vi "Parse_Limit_File.vi"(8 "error in":errorcluster, 11 "file path (dialog if empty)":path) -> (0 "error out":errorcluster, 1 "IncorrectString":string, 2 "AllThresholds":T1={"TC0"={"Enable"=FALSE, "LoErr"=0.0, "LoWarn"=0.0, "HiWarn"=0.0, "HiErr"=0.0, "RX?"=TRUE}, "TC1"={"Enable"=FALSE, "LoErr"=0.0, "LoWarn"=0.0, "HiWarn"=0.0, "HiErr"=0.0, "RX?"=TRUE}, "TC2"={"Enable"=FALSE, "LoErr"=0.0, "LoWarn"=0.0, "HiWarn"=0.0, "HiErr"=0.0, "RX?"=TRUE}, "TC3"={"Enable"=FALSE, "LoErr"=0.0, "LoWarn"=0.0, "HiWarn"=0.0, "HiErr"=0.0, "RX?"=TRUE}, "TC4"={"Enable"=FALSE, "LoErr"=0.0, "LoWarn"=0.0, "HiWarn"=0.0, "HiErr"=0.0, "RX?"=TRUE}, "TC5"={"Enable"=FALSE, "LoErr"=0.0, "LoWarn"=0.0, "HiWarn"=0.0, "HiErr"=0.0, "RX?"=TRUE}, "TC6"={"Enable"=FALSE, "LoErr"=0.0, "LoWarn"=0.0, "HiWarn"=0.0, "HiErr"=0.0, "RX?"=TRUE}, "TC7"={"Enable"=FALSE, "LoErr"=0.0, "LoWarn"=0.0, "HiWarn"=0.0, "HiErr"=0.0, "RX?"=TRUE}, "TC8"={"Enable"=FALSE, "LoErr"=0.0, "LoWarn"=0.0, "HiWarn"=0.0, "HiErr"=0.0, "RX?"=TRUE}, "TC9"={"Enable"=FALSE, "LoErr"=0.0, "LoWarn"=0.0, "HiWarn"=0.0, "HiErr"=0.0, "RX?"=TRUE}, "TC10"={"Enable"=FALSE, "LoErr"=0.0, "LoWarn"=0.0, "HiWarn"=0.0, "HiErr"=0.0, "RX?"=TRUE}, "TC11"={"Enable"=FALSE, "LoErr"=0.0, "LoWarn"=0.0, "HiWarn"=0.0, "HiErr"=0.0, "RX?"=TRUE}, "TC12"={"Enable"=FALSE, "LoErr"=0.0, "LoWarn"=0.0, "HiWarn"=0.0, "HiErr"=0.0, "RX?"=TRUE}, "TC13"={"Enable"=FALSE, "LoErr"=0.0, "LoWarn"=0.0, "HiWarn"=0.0, "HiErr"=0.0, "RX?"=TRUE}, "TC14"={"Enable"=FALSE, "LoErr"=0.0, "LoWarn"=0.0, "HiWarn"=0.0, "HiErr"=0.0, "RX?"=TRUE}, "TC15"={"Enable"=FALSE, "LoErr"=0.0, "LoWarn"=0.0, "HiWarn"=0.0, "HiErr"=0.0, "RX?"=TRUE}, "TC16"={"Enable"=FALSE, "LoErr"=0.0, "LoWarn"=0.0, "HiWarn"=0.0, "HiErr"=0.0, "RX?"=TRUE}, "TC17"={"Enable"=FALSE, "LoErr"=0.0, "LoWarn"=0.0, "HiWarn"=0.0, "HiErr"=0.0, "RX?"=TRUE}, "TC18"={"Enable"=FALSE, "LoErr"=0.0, "LoWarn"=0.0, "HiWarn"=0.0, "HiErr"=0.0, "RX?"=TRUE}, "TC19"={"Enable"=FALSE, "LoErr"=0.0, "LoWarn"=0.0, "HiWarn"=0.0, "HiErr"=0.0, "RX?"=TRUE}, "TC20"={"Enable"=FALSE, "LoErr"=0.0, "LoWarn"=0.0, "HiWarn"=0.0, "HiErr"=0.0, "RX?"=TRUE}, "AI0"={"Enable"=FALSE, "LoErr"=0.0, "LoWarn"=0.0, "HiWarn"=0.0, "HiErr"=0.0, "RX?"=TRUE}, "AI1"={"Enable"=FALSE, "LoErr"=0.0, "LoWarn"=0.0, "HiWarn"=0.0, "HiErr"=0.0, "RX?"=TRUE}, "AI2"={"Enable"=FALSE, "LoErr"=0.0, "LoWarn"=0.0, "HiWarn"=0.0, "HiErr"=0.0, "RX?"=TRUE}, "AI3"={"Enable"=FALSE, "LoErr"=0.0, "LoWarn"=0.0, "HiWarn"=0.0, "HiErr"=0.0, "RX?"=TRUE}, "AI4"={"Enable"=FALSE, "LoErr"=0.0, "LoWarn"=0.0, "HiWarn"=0.0, "HiErr"=0.0, "RX?"=TRUE}, "AI5"={"Enable"=FALSE, "LoErr"=0.0, "LoWarn"=0.0, "HiWarn"=0.0, "HiErr"=0.0, "RX?"=TRUE}, "AI6"={"Enable"=FALSE, "LoErr"=0.0, "LoWarn"=0.0, "HiWarn"=0.0, "HiErr"=0.0, "RX?"=TRUE}, "AI7"={"Enable"=FALSE, "LoErr"=0.0, "LoWarn"=0.0, "HiWarn"=0.0, "HiErr"=0.0, "RX?"=TRUE}, "AI16"={"Enable"=FALSE, "LoErr"=0.0, "LoWarn"=0.0, "HiWarn"=0.0, "HiErr"=0.0, "RX?"=TRUE}, "AI17"={"Enable"=FALSE, "LoErr"=0.0, "LoWarn"=0.0, "HiWarn"=0.0, "HiErr"=0.0, "RX?"=TRUE}, "AI18"={"Enable"=FALSE, "LoErr"=0.0, "LoWarn"=0.0, "HiWarn"=0.0, "HiErr"=0.0, "RX?"=TRUE}, "AI19"={"Enable"=FALSE, "LoErr"=0.0, "LoWarn"=0.0, "HiWarn"=0.0, "HiErr"=0.0, "RX?"=TRUE}, "AI20"={"Enable"=FALSE, "LoErr"=0.0, "LoWarn"=0.0, "HiWarn"=0.0, "HiErr"=0.0, "RX?"=TRUE}, "AI21"={"Enable"=FALSE, "LoErr"=0.0, "LoWarn"=0.0, "HiWarn"=0.0, "HiErr"=0.0, "RX?"=TRUE}, "AI22"={"Enable"=FALSE, "LoErr"=0.0, "LoWarn"=0.0, "HiWarn"=0.0, "HiErr"=0.0, "RX?"=TRUE}, "AI23"={"Enable"=FALSE, "LoErr"=0.0, "LoWarn"=0.0, "HiWarn"=0.0, "HiErr"=0.0, "RX?"=TRUE}})   [LabVIEW 2018]
uses:
  Controls/Clusts/AllThresholds.ctl
  Controls/Clusts/ThresholdAlarmLimits.ctl
  <vilib>/Utility/file.llb/Read Delimited Spreadsheet (string).vi
  <vilib>/Utility/file.llb/Read Delimited Spreadsheet (DBL).vi
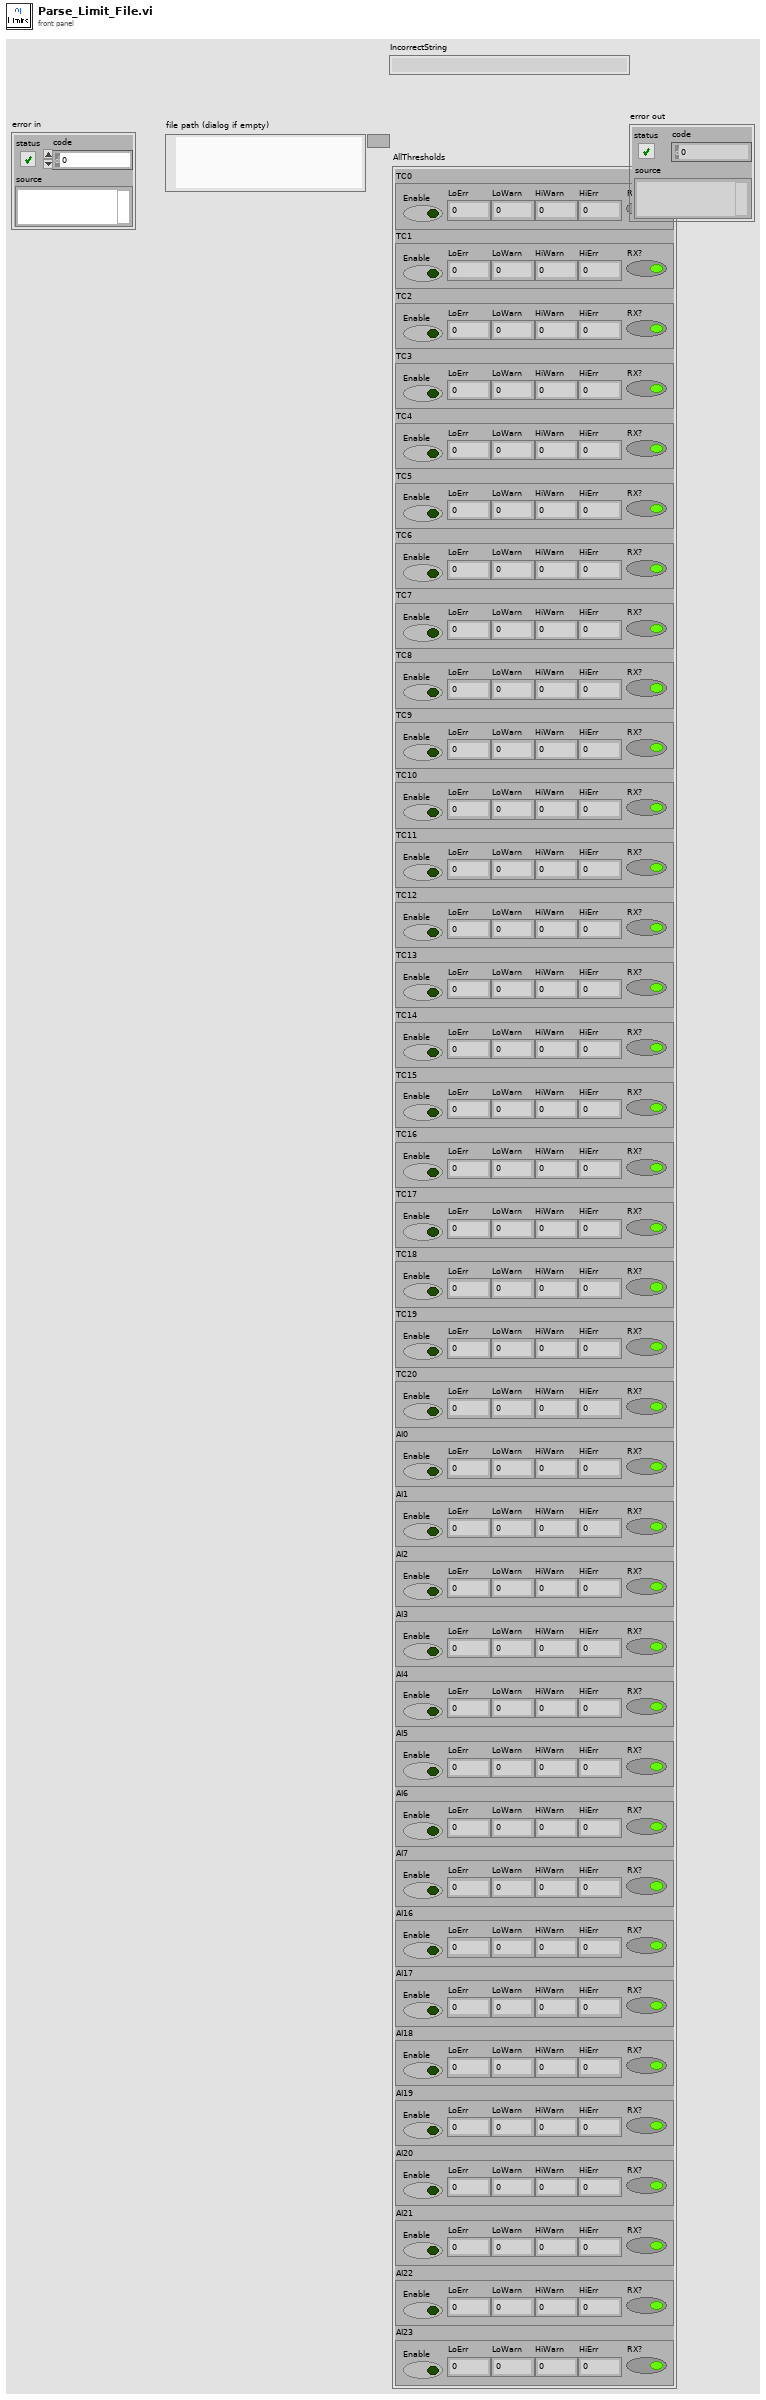
[diagram p1: front panel]
types:
  T1 = typedef "AllThresholds.ctl" = cluster{"TC0":T2, "TC1":T2, "TC2":T2, "TC3":T2, "TC4":T2, "TC5":T2, "TC6":T2, "TC7":T2, "TC8":T2, "TC9":T2, "TC10":T2, "TC11":T2, "TC12":T2, "TC13":T2, "TC14":T2, "TC15":T2, "TC16":T2, "TC17":T2, "TC18":T2, "TC19":T2, "TC20":T2, "AI0":T2, "AI1":T2, "AI2":T2, "AI3":T2, "AI4":T2, "AI5":T2, "AI6":T2, "AI7":T2, "AI16":T2, "AI17":T2, "AI18":T2, "AI19":T2, "AI20":T2, "AI21":T2, "AI22":T2, "AI23":T2}
  T2 = typedef "ThresholdAlarmLimits.ctl" = cluster{"Enable":bool, "LoErr":dbl, "LoWarn":dbl, "HiWarn":dbl, "HiErr":dbl, "RX?":bool}
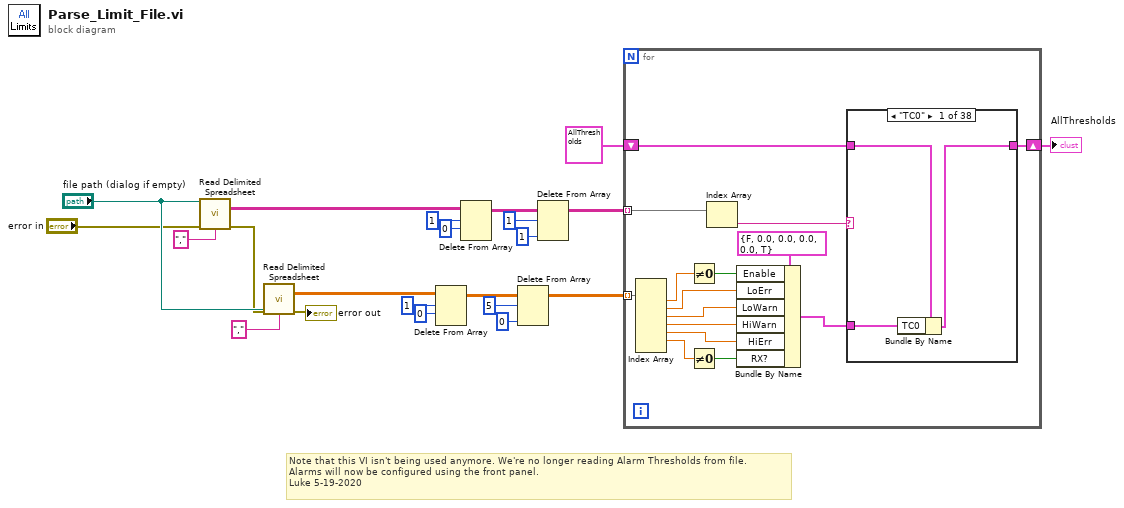
[diagram p0: block diagram]
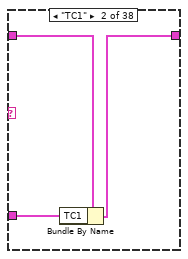
[diagram p2: hidden frame]
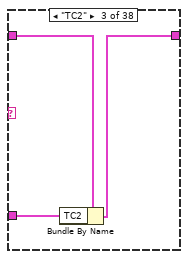
[diagram p3: hidden frame]
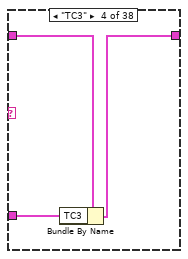
[diagram p4: hidden frame]
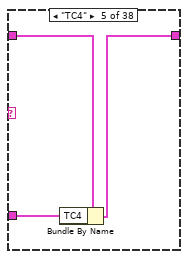
[diagram p5: hidden frame]
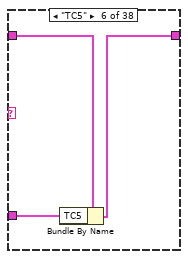
[diagram p6: hidden frame]
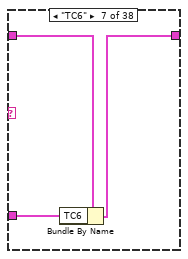
[diagram p7: hidden frame]
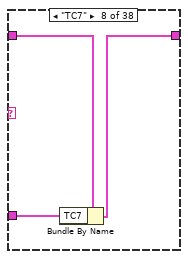
[diagram p8: hidden frame]
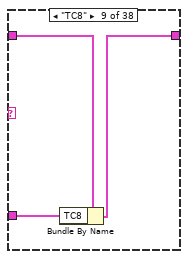
[diagram p9: hidden frame]
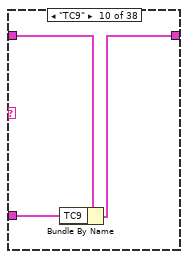
[diagram p10: hidden frame]
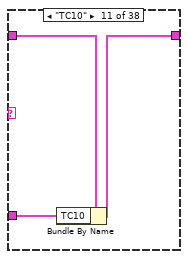
[diagram p11: hidden frame]
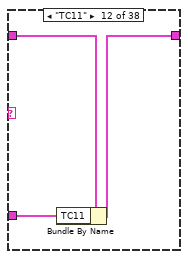
[diagram p12: hidden frame]
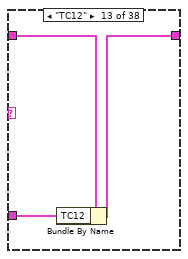
[diagram p13: hidden frame]
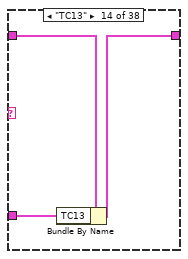
[diagram p14: hidden frame]
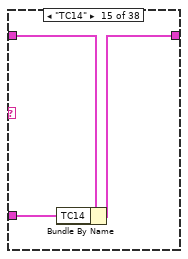
[diagram p15: hidden frame]
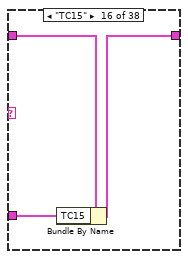
[diagram p16: hidden frame]
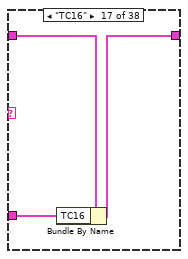
[diagram p17: hidden frame]
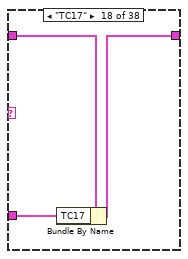
[diagram p18: hidden frame]
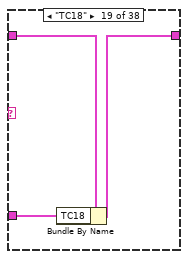
[diagram p19: hidden frame]
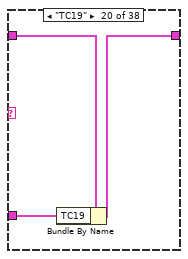
[diagram p20: hidden frame]
diagram:
  # "Note that this VI isn't being used anymore. We're no longer reading Alarm Thresholds from file.\nAlarms will now be configured using the front panel.\nLuke 5-19-2020"
  n1 = call-poly <vilib>:"Read Delimited Spreadsheet.vi"("file path (dialog if empty)"="file path (dialog if empty)", "error in (no error)"="error in", "delimiter (\\t)"="," ("delimiter (\\t)")) -> ("all rows"=w21:string[][], "error out"=w2:errorcluster)  [unwired: 7 in, 4 out]
  n2 = call-poly <vilib>:"Read Delimited Spreadsheet.vi"("file path (dialog if empty)"="file path (dialog if empty)", "error in (no error)"=w2, "delimiter (\\t)"="," ("delimiter (\\t)")) -> ("all rows"=w8:dbl[][], "error out"=→"error out":errorcluster)  [unwired: 7 in, 4 out]
  n3 = Delete From Array(array=w8, length=1, index (row)=0) -> (array with subset deleted=w12:dbl[][])  [unwired: 1 in, 1 out]
  n4 = Delete From Array(array=w21, length=1, index (row)=0) -> (array with subset deleted=w17:string[][])  [unwired: 1 in, 1 out]
  n5 = Delete From Array(array=w12, length=5, index (col)=0 ("disabled index (col)")) -> (array with subset deleted=w7:dbl[][])  [unwired: 1 in, 1 out]
  n6 = Delete From Array(array=w17, length=1, index (col)=1 ("disabled index (col)")) -> (array with subset deleted=w15:string[][])  [unwired: 1 in, 1 out]
  n7 = for {
    tunnel: w15 -> [w36] mode=indexing
    tunnel: w7 -> [w26] mode=indexing
    shift-right: [w35] -> w4
    shift-left: T1 {"TC0"={"Enable"=FALSE, "LoErr"=0.0, "LoWarn"=0.0, "HiWarn"=0.0, "HiErr"=0.0, "RX?"=TRUE}, "TC1"={"Enable"=FALSE, "LoErr"=0.0, "LoWarn"=0.0, "HiWarn"=0.0, "HiErr"=0.0, "RX?"=TRUE}, "TC2"={"Enable"=FALSE, "LoErr"=0.0, "LoWarn"=0.0, "HiWarn"=0.0, "HiErr"=0.0, "RX?"=TRUE}, "TC3"={"Enable"=FALSE, "LoErr"=0.0, "LoWarn"=0.0, "HiWarn"=0.0, "HiErr"=0.0, "RX?"=TRUE}, "TC4"={"Enable"=FALSE, "LoErr"=0.0, "LoWarn"=0.0, "HiWarn"=0.0, "HiErr"=0.0, "RX?"=TRUE}, "TC5"={"Enable"=FALSE, "LoErr"=0.0, "LoWarn"=0.0, "HiWarn"=0.0, "HiErr"=0.0, "RX?"=TRUE}, "TC6"={"Enable"=FALSE, "LoErr"=0.0, "LoWarn"=0.0, "HiWarn"=0.0, "HiErr"=0.0, "RX?"=TRUE}, "TC7"={"Enable"=FALSE, "LoErr"=0.0, "LoWarn"=0.0, "HiWarn"=0.0, "HiErr"=0.0, "RX?"=TRUE}, "TC8"={"Enable"=FALSE, "LoErr"=0.0, "LoWarn"=0.0, "HiWarn"=0.0, "HiErr"=0.0, "RX?"=TRUE}, "TC9"={"Enable"=FALSE, "LoErr"=0.0, "LoWarn"=0.0, "HiWarn"=0.0, "HiErr"=0.0, "RX?"=TRUE}, "TC10"={"Enable"=FALSE, "LoErr"=0.0, "LoWarn"=0.0, "HiWarn"=0.0, "HiErr"=0.0, "RX?"=TRUE}, "TC11"={"Enable"=FALSE, "LoErr"=0.0, "LoWarn"=0.0, "HiWarn"=0.0, "HiErr"=0.0, "RX?"=TRUE}, "TC12"={"Enable"=FALSE, "LoErr"=0.0, "LoWarn"=0.0, "HiWarn"=0.0, "HiErr"=0.0, "RX?"=TRUE}, "TC13"={"Enable"=FALSE, "LoErr"=0.0, "LoWarn"=0.0, "HiWarn"=0.0, "HiErr"=0.0, "RX?"=TRUE}, "TC14"={"Enable"=FALSE, "LoErr"=0.0, "LoWarn"=0.0, "HiWarn"=0.0, "HiErr"=0.0, "RX?"=TRUE}, "TC15"={"Enable"=FALSE, "LoErr"=0.0, "LoWarn"=0.0, "HiWarn"=0.0, "HiErr"=0.0, "RX?"=TRUE}, "TC16"={"Enable"=FALSE, "LoErr"=0.0, "LoWarn"=0.0, "HiWarn"=0.0, "HiErr"=0.0, "RX?"=TRUE}, "TC17"={"Enable"=FALSE, "LoErr"=0.0, "LoWarn"=0.0, "HiWarn"=0.0, "HiErr"=0.0, "RX?"=TRUE}, "TC18"={"Enable"=FALSE, "LoErr"=0.0, "LoWarn"=0.0, "HiWarn"=0.0, "HiErr"=0.0, "RX?"=TRUE}, "TC19"={"Enable"=FALSE, "LoErr"=0.0, "LoWarn"=0.0, "HiWarn"=0.0, "HiErr"=0.0, "RX?"=TRUE}, "TC20"={"Enable"=FALSE, "LoErr"=0.0, "LoWarn"=0.0, "HiWarn"=0.0, "HiErr"=0.0, "RX?"=TRUE}, "AI0"={"Enable"=FALSE, "LoErr"=0.0, "LoWarn"=0.0, "HiWarn"=0.0, "HiErr"=0.0, "RX?"=TRUE}, "AI1"={"Enable"=FALSE, "LoErr"=0.0, "LoWarn"=0.0, "HiWarn"=0.0, "HiErr"=0.0, "RX?"=TRUE}, "AI2"={"Enable"=FALSE, "LoErr"=0.0, "LoWarn"=0.0, "HiWarn"=0.0, "HiErr"=0.0, "RX?"=TRUE}, "AI3"={"Enable"=FALSE, "LoErr"=0.0, "LoWarn"=0.0, "HiWarn"=0.0, "HiErr"=0.0, "RX?"=TRUE}, "AI4"={"Enable"=FALSE, "LoErr"=0.0, "LoWarn"=0.0, "HiWarn"=0.0, "HiErr"=0.0, "RX?"=TRUE}, "AI5"={"Enable"=FALSE, "LoErr"=0.0, "LoWarn"=0.0, "HiWarn"=0.0, "HiErr"=0.0, "RX?"=TRUE}, "AI6"={"Enable"=FALSE, "LoErr"=0.0, "LoWarn"=0.0, "HiWarn"=0.0, "HiErr"=0.0, "RX?"=TRUE}, "AI7"={"Enable"=FALSE, "LoErr"=0.0, "LoWarn"=0.0, "HiWarn"=0.0, "HiErr"=0.0, "RX?"=TRUE}, "AI16"={"Enable"=FALSE, "LoErr"=0.0, "LoWarn"=0.0, "HiWarn"=0.0, "HiErr"=0.0, "RX?"=TRUE}, "AI17"={"Enable"=FALSE, "LoErr"=0.0, "LoWarn"=0.0, "HiWarn"=0.0, "HiErr"=0.0, "RX?"=TRUE}, "AI18"={"Enable"=FALSE, "LoErr"=0.0, "LoWarn"=0.0, "HiWarn"=0.0, "HiErr"=0.0, "RX?"=TRUE}, "AI19"={"Enable"=FALSE, "LoErr"=0.0, "LoWarn"=0.0, "HiWarn"=0.0, "HiErr"=0.0, "RX?"=TRUE}, "AI20"={"Enable"=FALSE, "LoErr"=0.0, "LoWarn"=0.0, "HiWarn"=0.0, "HiErr"=0.0, "RX?"=TRUE}, "AI21"={"Enable"=FALSE, "LoErr"=0.0, "LoWarn"=0.0, "HiWarn"=0.0, "HiErr"=0.0, "RX?"=TRUE}, "AI22"={"Enable"=FALSE, "LoErr"=0.0, "LoWarn"=0.0, "HiWarn"=0.0, "HiErr"=0.0, "RX?"=TRUE}, "AI23"={"Enable"=FALSE, "LoErr"=0.0, "LoWarn"=0.0, "HiWarn"=0.0, "HiErr"=0.0, "RX?"=TRUE}} ("AllThresholds") -> [w34]
    n8 = Index Array(array=w26) -> (element #1=w23:dbl, element #2=w28:dbl, element #3=w29:dbl, element #4=w30:dbl, element #5=w31:dbl, element #6=w32:dbl)  [unwired: 7 in, 1 out]
    n9 = Not Equal To 0?(x=w23) -> (x != 0?=w24:bool)
    n10 = Not Equal To 0?(x=w32) -> (x != 0?=w33:bool)
    n11 = Index Array(array=w36) -> (element=w37:string)  [unwired: 1 in]
    n12 = Bundle By Name(cluster=T2 {"Enable"=FALSE, "LoErr"=0.0, "LoWarn"=0.0, "HiWarn"=0.0, "HiErr"=0.0, "RX?"=TRUE} ("TC0"), "Enable"=w24, "LoErr"=w28, "LoWarn"=w29, "HiWarn"=w30, "HiErr"=w31, "RX?"=w33) -> (w25:T2)
    n13 = case shown="\"TC0\"" w37 {
      selector: w37 -> [_ _ _ _ _ _ _ _ _ _ _ _ _ _ _ _ _ _ _ _ _ _ _ _ _ _ _ _ _ _ _ _ _ _ _ _ _ w149]
      tunnel: [w39 w42 w45 w48 w51 w54 w57 w60 w63 w66 w69 w72 w75 w78 w81 w84 w87 w90 w93 w96 w99 w102 w105 w108 w111 w114 w117 w120 w123 w126 w129 w132 w135 w138 w141 w144 w147 w150] -> w35
      tunnel: w34 -> [w40 w43 w46 w49 w52 w55 w58 w61 w64 w67 w70 w73 w76 w79 w82 w85 w88 w91 w94 w97 w100 w103 w106 w109 w112 w115 w118 w121 w124 w127 w130 w133 w136 w139 w142 w145 w148 w150]
      tunnel: w25 -> [w38 w41 w44 w47 w50 w53 w56 w59 w62 w65 w68 w71 w74 w77 w80 w83 w86 w89 w92 w95 w98 w101 w104 w107 w110 w113 w116 w119 w122 w125 w128 w131 w134 w137 w140 w143 w146 _]
      frame "TC0" {
        n14 = Bundle By Name(cluster=w40, "TC0"=w38) -> (w39:T1)
      }
      frame "TC1" {
        n15 = Bundle By Name(cluster=w43, "TC1"=w41) -> (w42:T1)
      }
      frame "TC2" {
        n16 = Bundle By Name(cluster=w46, "TC2"=w44) -> (w45:T1)
      }
      frame "TC3" {
        n17 = Bundle By Name(cluster=w49, "TC3"=w47) -> (w48:T1)
      }
      frame "TC4" {
        n18 = Bundle By Name(cluster=w52, "TC4"=w50) -> (w51:T1)
      }
      frame "TC5" {
        n19 = Bundle By Name(cluster=w55, "TC5"=w53) -> (w54:T1)
      }
      frame "TC6" {
        n20 = Bundle By Name(cluster=w58, "TC6"=w56) -> (w57:T1)
      }
      frame "TC7" {
        n21 = Bundle By Name(cluster=w61, "TC7"=w59) -> (w60:T1)
      }
      frame "TC8" {
        n22 = Bundle By Name(cluster=w64, "TC8"=w62) -> (w63:T1)
      }
      frame "TC9" {
        n23 = Bundle By Name(cluster=w67, "TC9"=w65) -> (w66:T1)
      }
      frame "TC10" {
        n24 = Bundle By Name(cluster=w70, "TC10"=w68) -> (w69:T1)
      }
      frame "TC11" {
        n25 = Bundle By Name(cluster=w73, "TC11"=w71) -> (w72:T1)
      }
      frame "TC12" {
        n26 = Bundle By Name(cluster=w76, "TC12"=w74) -> (w75:T1)
      }
      frame "TC13" {
        n27 = Bundle By Name(cluster=w79, "TC13"=w77) -> (w78:T1)
      }
      frame "TC14" {
        n28 = Bundle By Name(cluster=w82, "TC14"=w80) -> (w81:T1)
      }
      frame "TC15" {
        n29 = Bundle By Name(cluster=w85, "TC15"=w83) -> (w84:T1)
      }
      frame "TC16" {
        n30 = Bundle By Name(cluster=w88, "TC16"=w86) -> (w87:T1)
      }
      frame "TC17" {
        n31 = Bundle By Name(cluster=w91, "TC17"=w89) -> (w90:T1)
      }
      frame "TC18" {
        n32 = Bundle By Name(cluster=w94, "TC18"=w92) -> (w93:T1)
      }
      frame "TC19" {
        n33 = Bundle By Name(cluster=w97, "TC19"=w95) -> (w96:T1)
      }
      frame "TC20" {
        n34 = Bundle By Name(cluster=w100, "TC20"=w98) -> (w99:T1)
      }
      frame "AI0" {
        n35 = Bundle By Name(cluster=w103, "AI0"=w101) -> (w102:T1)
      }
      frame "AI1" {
        n36 = Bundle By Name(cluster=w106, "AI1"=w104) -> (w105:T1)
      }
      frame "AI2" {
        n37 = Bundle By Name(cluster=w109, "AI2"=w107) -> (w108:T1)
      }
      frame "AI3" {
        n38 = Bundle By Name(cluster=w112, "AI3"=w110) -> (w111:T1)
      }
      frame "AI4" {
        n39 = Bundle By Name(cluster=w115, "AI4"=w113) -> (w114:T1)
      }
      frame "AI5" {
        n40 = Bundle By Name(cluster=w118, "AI5"=w116) -> (w117:T1)
      }
      frame "AI6" {
        n41 = Bundle By Name(cluster=w121, "AI6"=w119) -> (w120:T1)
      }
      frame "AI7" {
        n42 = Bundle By Name(cluster=w124, "AI7"=w122) -> (w123:T1)
      }
      frame "AI16" {
        n43 = Bundle By Name(cluster=w127, "AI16"=w125) -> (w126:T1)
      }
      frame "AI17" {
        n44 = Bundle By Name(cluster=w130, "AI17"=w128) -> (w129:T1)
      }
      frame "AI18" {
        n45 = Bundle By Name(cluster=w133, "AI18"=w131) -> (w132:T1)
      }
      frame "AI19" {
        n46 = Bundle By Name(cluster=w136, "AI19"=w134) -> (w135:T1)
      }
      frame "AI20" {
        n47 = Bundle By Name(cluster=w139, "AI20"=w137) -> (w138:T1)
      }
      frame "AI21" {
        n48 = Bundle By Name(cluster=w142, "AI21"=w140) -> (w141:T1)
      }
      frame "AI22" {
        n49 = Bundle By Name(cluster=w145, "AI22"=w143) -> (w144:T1)
      }
      frame "AI23" {
        n50 = Bundle By Name(cluster=w148, "AI23"=w146) -> (w147:T1)
      }
      frame Default {
        "IncorrectString" <- w149
      }
    }
  }
  "AllThresholds" <- w4
